vi "Read Discovery Service Key File.vi"(8 "error in (no error)":errorcluster, 11 "key file path":path) -> (0 "error out":errorcluster, 3 "key json":string)   [LabVIEW 2020, in "LoadRegulation.lvlib"]
uses:
  LoadRegulation.lvlib
  kernel32.dll
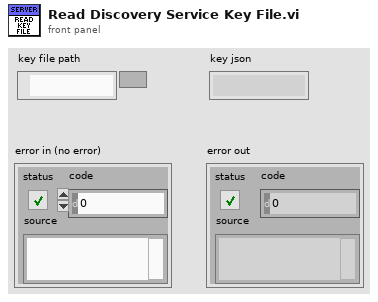
[diagram p1: front panel]
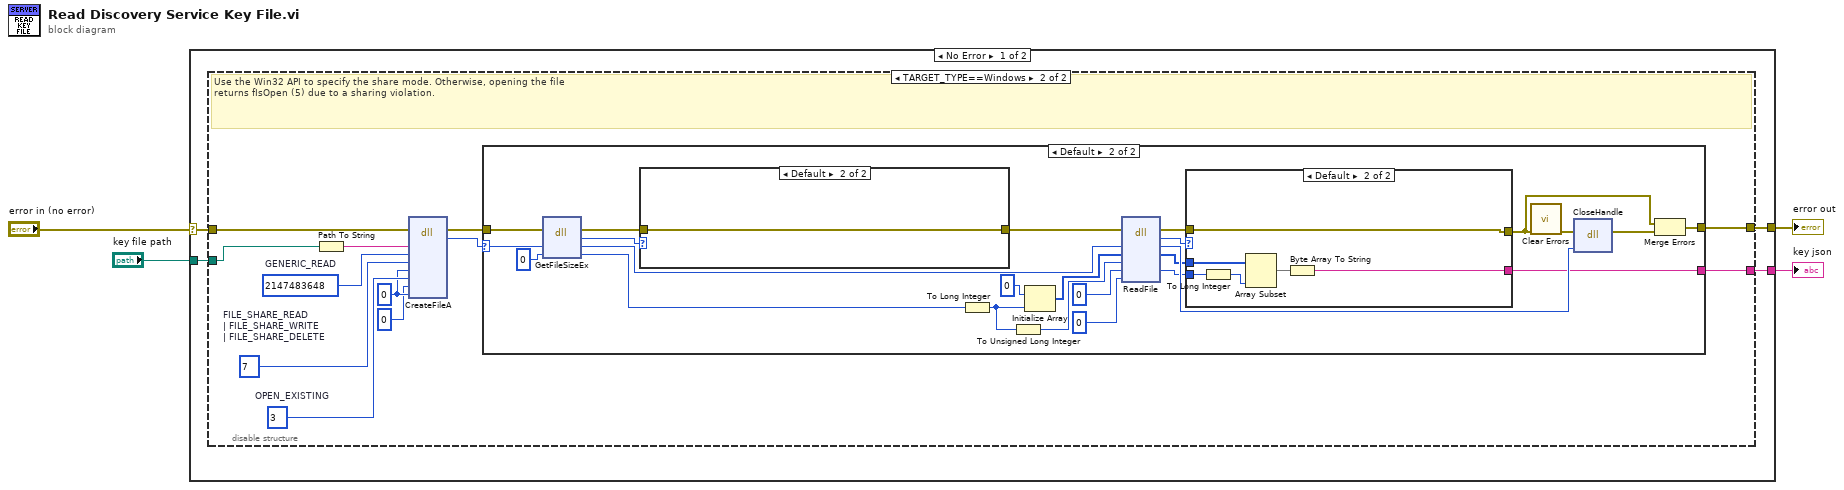
[diagram p0: block diagram]
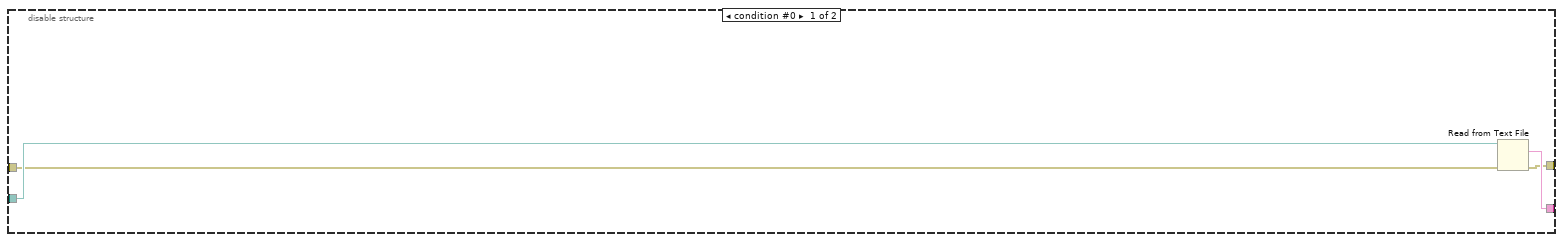
[diagram p2: hidden frame]
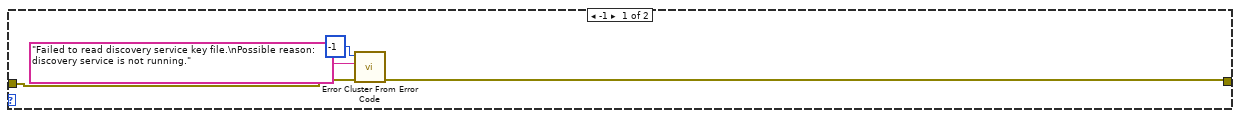
[diagram p3: hidden frame]
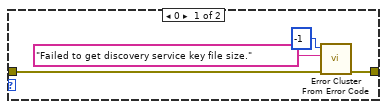
[diagram p4: hidden frame]
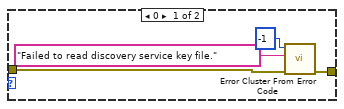
[diagram p5: hidden frame]
diagram:
  n1 = case shown="No Error" "error in (no error)" {
    selector: "error in (no error)" -> [w5 w68]
    tunnel: [w8 w68] -> w4
    tunnel: [w7 _] -> w3
    tunnel: "key file path" -> [w6 _]
    frame No Error {
      n2 = disable-structure shown="TARGET_TYPE==Windows" {
        disable-tunnel: w6 -> [w12 w16]
        disable-tunnel: w5 -> [w11 w15]
        disable-tunnel: [w10 w14] -> w7
        disable-tunnel: [w9 w13] -> w8
        frame condition #0 {
          n3 = Read from Text File(file (use dialog)=w12, error in=w11) -> (text=w10:string, error out=w9:errorcluster)  [unwired: 2 in, 2 out]
        }
        frame condition #1 (active) {
          w20 = i64 0 ("lpSecurityAttributes")
          w21 = u32 3  # OPEN_EXISTING
          w22 = u32 7  # FILE_SHARE_READ  | FILE_SHARE_WRITE  | FILE_SHARE_DELETE
          w23 = u32 2147483648  # GENERIC_READ
          # "Use the Win32 API to specify the share mode. Otherwise, opening the file\nreturns fIsOpen (5) due to a sharing violation."
          n4 = Path To String(path=w16) -> (string=w24:string)
          n5 = dll-call lib="kernel32.dll" fn="CreateFileA"(error in=w15, "lpFileName"=w24, "dwDesiredAccess"=w23, "dwShareMode"=w22, "lpSecurityAttributes"=w20, "dwCreationDisposition"=w21, "dwFlagsAndAttributes"=u32 0, "hTemplateFile"=w20) -> (error out=w17:errorcluster, "return type"=w18:i64)  [unwired: 9 in, 1 out]
          n6 = case shown="Default" w18 {
            selector: w18 -> [_ w37]
            tunnel: w17 -> [w26 w35]
            tunnel: [w25 w46] -> w13
            tunnel: [_ w40] -> w14
            frame -1 {
              n7 = call <vilib>:"Error Cluster From Error Code.vi"("error in (no error)"=w26, "error message (\"\")"="Failed to read discovery service key file.\nPossible reason: discovery service is not running." ("error message (\"\")"), "error code (0)"=-1) -> ("error out"=w25:errorcluster)  [unwired: 6 in]
            }
            frame Default {
              n8 = dll-call lib="kernel32.dll" fn="GetFileSizeEx"(error in=w35, "hFile"=w37, "lpFileSize"=i64 0) -> (error out=w32:errorcluster, "return type"=w31:i32, "hFile"=w36:i64, "lpFileSize"=w33:i64)  [unwired: 2 in, 1 out]
              n9 = case shown="Default" w31 {
                tunnel: w32 -> [w54 w57]
                tunnel: [w53 w57] -> w30
                frame 0 {
                  n10 = call <vilib>:"Error Cluster From Error Code.vi"("error in (no error)"=w54, "error message (\"\")"="Failed to get discovery service key file size." ("error message (\"\")"), "error code (0)"=-1) -> ("error out"=w53:errorcluster)  [unwired: 6 in]
                }
                frame Default {
                }
              }
              n11 = To Long Integer(number=w33) -> (32bit integer=w29:i32)
              n12 = To Unsigned Long Integer(number=w29) -> (unsigned 32bit integer=w51:u32)
              n13 = Initialize Array(u8 0, w29) -> (w50:u8[])
              n14 = dll-call lib="kernel32.dll" fn="ReadFile"(error in=w30, "hFile"=w36, "lpBuffer"=w50, "nNumberOfBytesToRead"=w51, "lpNumberOfBytesRead"=u32 0, "lpOverlapped"=i64 0) -> (error out=w43:errorcluster, "return type"=w44:i32, "hFile"=w45:i64, "lpBuffer"=w42:u8[], "lpNumberOfBytesRead"=w41:u32)  [unwired: 4 in, 1 out]
              n15 = case shown="Default" w44 {
                tunnel: w43 -> [w59 w63]
                tunnel: [w58 w63] -> w38
                tunnel: w42 -> [_ w67]
                tunnel: w41 -> [_ w66]
                tunnel: [_ w62] -> w40
                frame 0 {
                  n16 = call <vilib>:"Error Cluster From Error Code.vi"("error in (no error)"=w59, "error message (\"\")"="Failed to read discovery service key file." ("error message (\"\")"), "error code (0)"=-1) -> ("error out"=w58:errorcluster)  [unwired: 6 in]
                }
                frame Default {
                  n17 = To Long Integer(number=w66) -> (32bit integer=w65:i32)
                  n18 = Array Subset(array=w67, length=w65) -> (w64:u8[])  [unwired: 1 in]
                  n19 = Byte Array To String(unsigned byte array=w64) -> (string=w62:string)
                }
              }
              n20 = call <vilib>:"Clear Errors.vi"("error in (no error)"=w38) -> ("error out"=w39:errorcluster)  [unwired: 5 in, 1 out]
              n21 = dll-call lib="kernel32.dll" fn="CloseHandle"(error in=w39, "hObject"=w45) -> (error out=w47:errorcluster)  [unwired: 4 in, 1 out]
              n22 = Merge Errors(w38, w47) -> (w46:errorcluster)
            }
          }
        }
      }
    }
    frame Error {
    }
  }
  "error out" <- w4
  "key json" <- w3
